vi "Get Array Type.vi"(8 "error in (no error)":errorcluster, 11 "Abs_Time 1D.lvclass":refnum<class "Abs_Waveform 1D.lvclass">) -> (0 "error out":errorcluster, 2 "Type":T1, 3 "Abs_Time 1D.lvclass":refnum<class "Abs_Waveform 1D.lvclass">)   [LabVIEW 2021, in "Abs_Waveform 1D.lvclass"]
uses:
  Abs_Waveform 1D.lvclass
  <vilib>/Utility/Data Type/Type Definitions/Data Type.ctl
  <vilib>/Utility/Data Type/NI_Data Type.lvlib
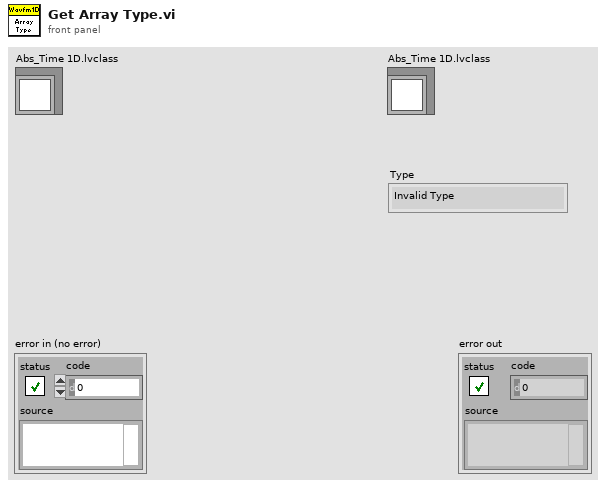
[diagram p1: front panel]
types:
  T1 = typedef "NI_Data Type.lvlib/Data Type.ctl" = enum8{"Invalid Type", "Void", "I8", "I16", "I32", "I64", "U8", "U16", "U32", "U64", "Single Float", "Double Float", "Extended Float", "Single Complex", "Double Complex", "Extended Complex", "Enum U8", "Enum U16", "Enum U32", "Enum U64", "Single Float With Unit", "Double Float With Unit", "Extended Float With Unit", "Single Complex with Unit", "Double Complex with Unit", "Extended Complex with Unit", "Boolean", "String", "Path", "Picture", "Tag", "Array", "Cluster", "Variant", "LV Variant", "Waveform", "Timestamp", "Digital Waveform", "Digital Data", "ExpressData", "Refnum", "External Data", "VI", "Poly VI", "LabVIEW Class Instance", "Fixed Point", "Set Collection", "Map Collection"}
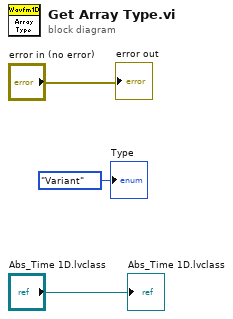
[diagram p0: block diagram]
diagram:
  "error out" <- "error in (no error)"
  "Type" <- Data_Type."Variant" ("Type")
  "Abs_Time 1D.lvclass" <- "Abs_Time 1D.lvclass"
